vi "get_this_state.vi"(8 "error in (no error)":errorcluster, 11 "Lua in":refnum<class "Lua.lvclass">) -> (0 "error out":errorcluster, 2 "this state":refnum<data-value>, 3 "Lua out":refnum<class "Lua.lvclass">)   [LabVIEW 2020, in "Lua for LabVIEW.lvlib" / "Lua.lvclass"]
uses:
  Lua.lvclass
  Lua.lvclass/Lua.ctl
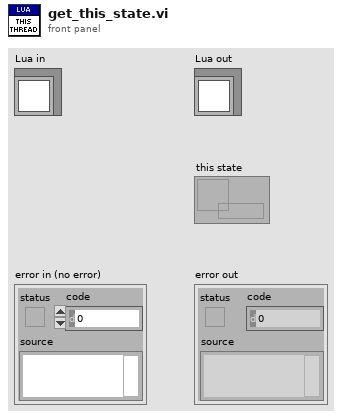
[diagram p1: front panel]
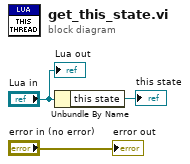
[diagram p0: block diagram]
diagram:
  n1 = Unbundle By Name("Lua in") -> ("this state"=→"this state":refnum<data-value>)
  "error out" <- "error in (no error)"
  "Lua out" <- "Lua in"
